vi "Arduino Hello World Test Program.vi"() -> ()   [LabVIEW 2021, in "FW Arduino Control.lvclass"]
uses:
  FW Arduino Control.lvclass
  2f98032c-9b9c-4006-b353-488e19d3a6eb.vi
panel:
  out "reset response":string
  in  "Stop":bool
  out "pos":i32(graph)
  out "response":string
  in  "VISA resource name":refnum<visa-resource-name>="COM9"
  in  "Curr Pos":i32
  in  "Target Pos":i32
  in  "Filter Wheel (0:n-1)":i32
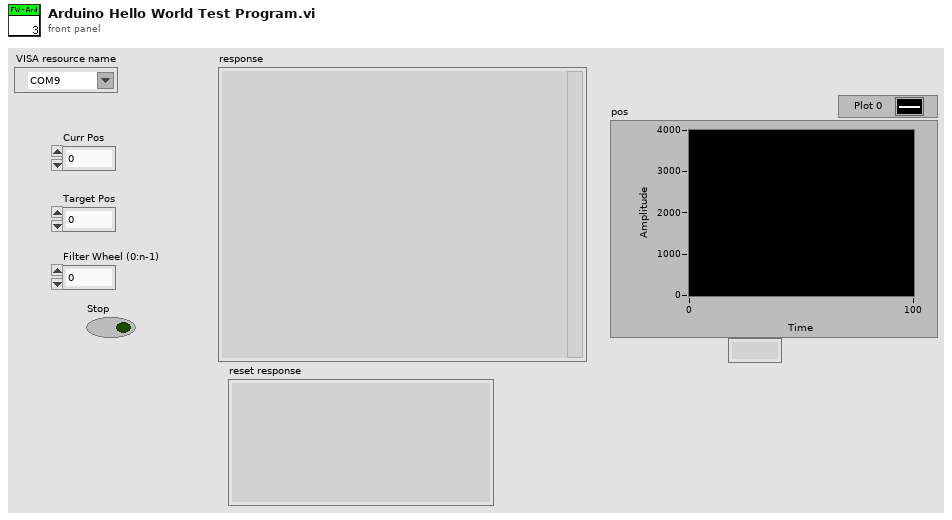
[diagram p1: front panel]
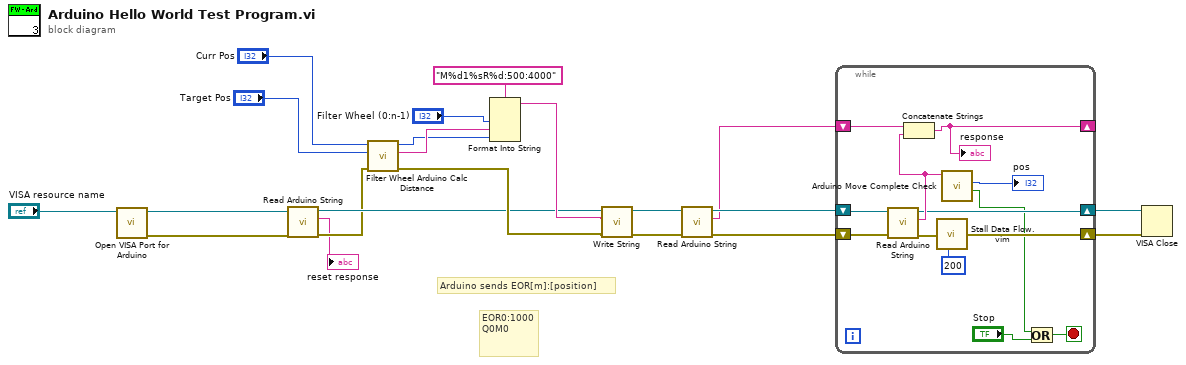
[diagram p0: block diagram]
diagram:
  # "EOR0:1000\nQ0M0"
  # "Arduino sends EOR[m]:[position]"
  n1 = call "Open VISA Port for Arduino.vi"("VISA resource name"="VISA resource name") -> ("error out"=w1:errorcluster, "VISA resource name out"=w2:refnum<visa-resource-name>)  [unwired: 9 in]
  n2 = call "Read Arduino String.vi"("error in (no error)"=w1, "reference"=w2) -> ("error out"=w6:errorcluster, "response"=→"reset response":string, "reference out"=w7:refnum<visa-resource-name>)  [unwired: 7 in]
  n3 = call "Filter Wheel Arduino Calc Distance.vi"("error in (no error)"=w6, "To Position"="Target Pos", "From Pos"="Curr Pos") -> ("error out"=w14:errorcluster, "Direction"=w20:string, "Counts"=w19:u32)  [unwired: 6 in]
  n4 = Format Into String(format string="M%d1%sR%d:500:4000", "Filter Wheel (0:n-1)", w20, w19) -> (resulting string=w15:string)  [unwired: 2 in, 1 out]
  n5 = call "Write String.vi"("error in (no error)"=w14, "String"=w15, "VISA resource name"=w7) -> ("error out"=w8:errorcluster, "VISA resource name out"=w9:refnum<visa-resource-name>)  [unwired: 7 in]
  n6 = call "Read Arduino String.vi"("error in (no error)"=w8, "reference"=w9) -> ("error out"=w12:errorcluster, "response"=w4:string, "reference out"=w13:refnum<visa-resource-name>)  [unwired: 7 in]
  n7 = while {
    shift-right: [w25] -> w10
    shift-left: w13 -> [w31]
    shift-right: [w33] -> w3
    shift-left: w12 -> [w29]
    shift-right: [w26] -> _
    shift-left: w4 -> [w27]
    stop <- w23 stop-if-true
    n8 = call "Read Arduino String.vi"("error in (no error)"=w29, "reference"=w31) -> ("error out"=w30:errorcluster, "response"=w28:string, "reference out"=w25:refnum<visa-resource-name>)  [unwired: 7 in]
    n9 = Concatenate Strings(w27, w28) -> (w26:string)
    "response" <- w26
    n10 = call "Stall Data Flow.vim"("value in"=w30, "milliseconds to wait"=u32 200) -> ("value out"=w33:errorcluster)  [unwired: 1 out]
    n11 = call "Arduino Move Complete Check.vi"("input string"=w28) -> ("Complete?"=w22:bool, "position"=→"pos":i32)  [unwired: 8 in, 1 out]
    n12 = Or(x=w22, y="Stop") -> (x .or. y?=w23:bool)
  }
  n13 = VISA Close(VISA resource name=w10, error in (no error)=w3) -> ()  [unwired: 1 out]
